vi "Data Format.vi"() -> ()   [LabVIEW 2012]
panel:
  in  "Cap_Data":string[][](table)=[["0x02", "3.76992", "0x02", "3.77728"], ["0x02", "3.78382", "0x00", "-8.19200"], ["0x02", "3.94961", "0x02", "3.76741"], ["0x02", "4.54733", "0x02", "4.63408"], ["0x02", "3.84893", "0x02", "3.82712"], ["0x02", "3.80094", "0x02", "3.80246"], ["0x02", "3.79069", "0x02", "3.74972"], ["0x02", "3.80074", "0x02", "3.79936"], ["0x02", "4.04241", "0x02", "3.22665"], ["0x02", "3.79415", "0x02", "3.76417"], ["0x02", "3.79553", "0x02", "3.77940"], ["0x02", "1.03695", "0x02", "1.03735"], ["0x02", "3.80021", "0x02", "3.77078"], ["0x02", "4.65608", "0x02", "4.70829"], ["0x02", "3.74688", "0x02", "3.75749"], ["0x02", "3.81169", "0x02", "3.79781"]]
  out "output array":string[](array[string])
  out "Data Output":string[][](table)
  out "Reg3&4 2":string[](array[string])
  out "Reg1&2 2":string[](array[string])
  out "Reg3&4":string[](array[string])
  out "Reg1&2":string[](array[string])
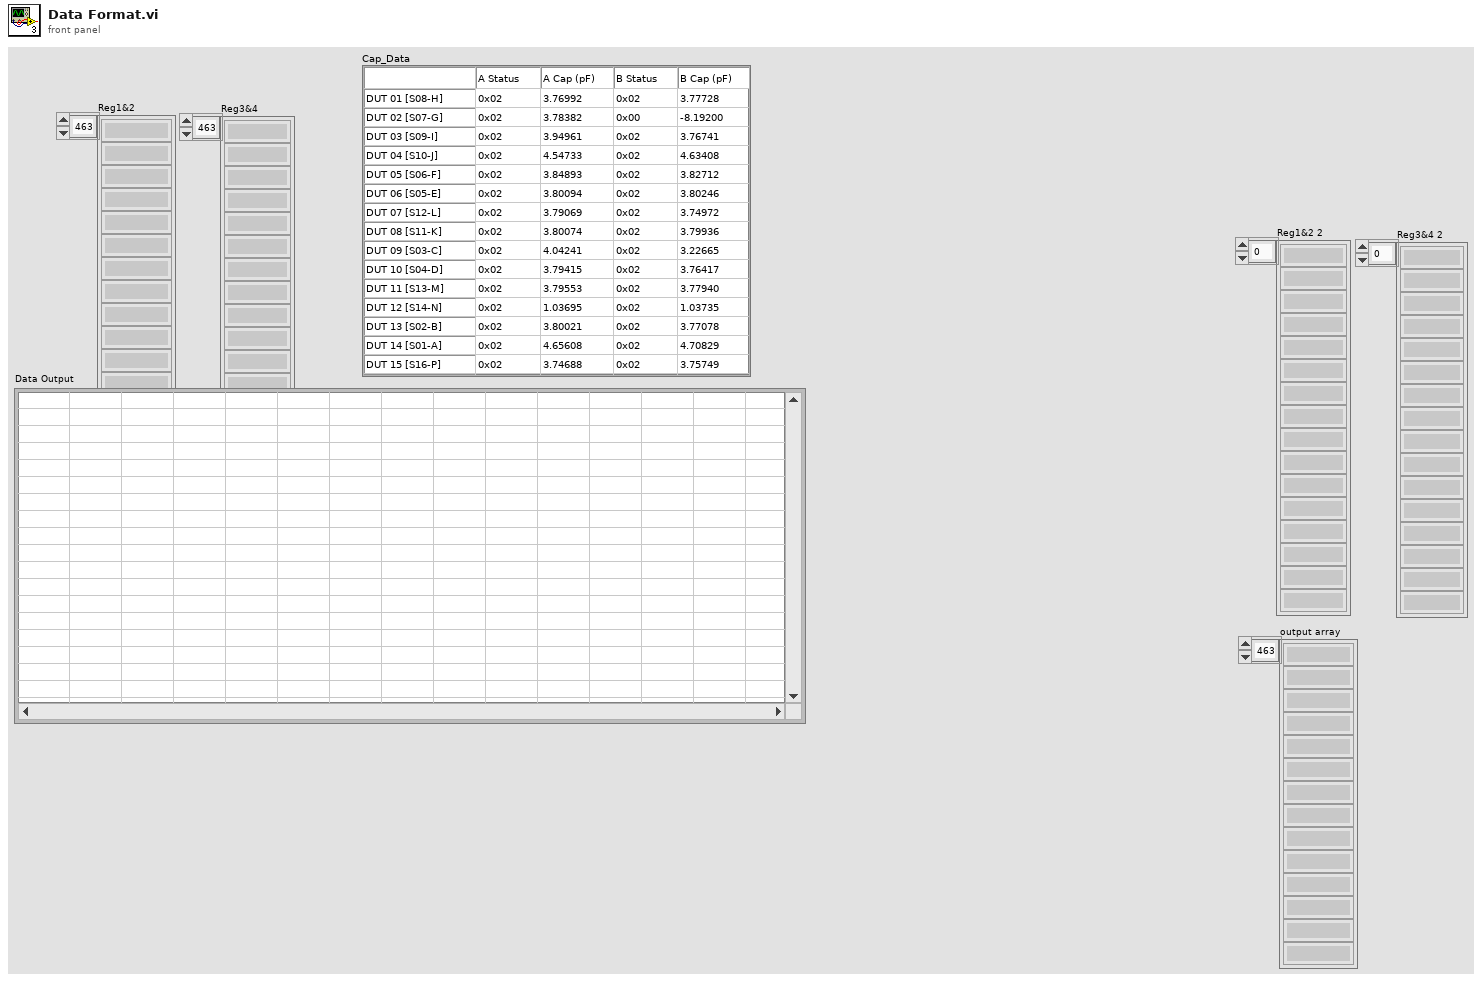
[diagram p1: front panel]
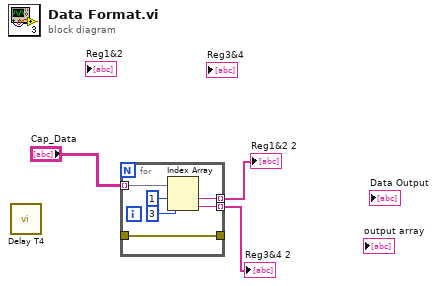
[diagram p0: block diagram]
diagram:
  n1 = call "Delay T4.vi"() -> ()  [unwired: 11 in, 1 out]
  n2 = for {
    tunnel: "Cap_Data" -> [w11] mode=indexing
    tunnel: [w12] -> w5
    tunnel: [w12] -> w4
    tunnel: [w8] -> w2 mode=indexing
    tunnel: [w7] -> w3 mode=indexing
    n3 = Index Array(array=w11, index #1=1 ("index"), index #2=3 ("index")) -> (element #1=w8:string, element #2=w7:string)
  }
  "Reg1&2 2" <- w2
  "Reg3&4 2" <- w3
